vi "String_to_Pathname.vi"(1 "Input String":string) -> (0 "path":path)   [LabVIEW 2014]
uses:
  Globals/Preference_global.vi
  Globals/Constants_global.vi
panel:
  out "size(s)":i32
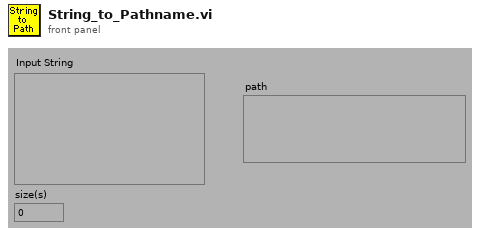
[diagram p1: front panel]
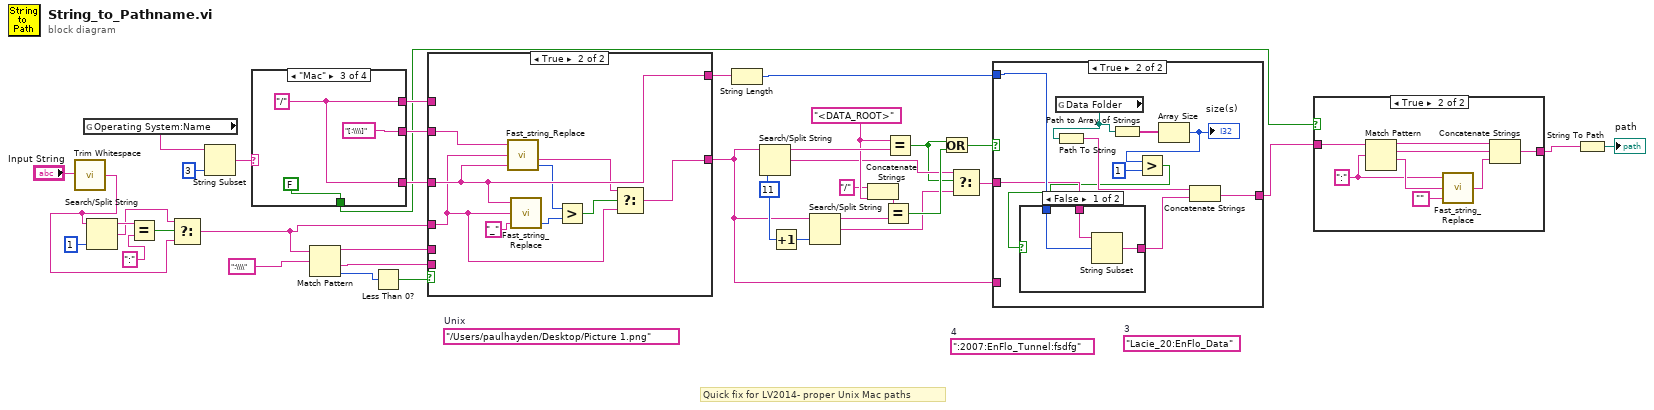
[diagram p0: block diagram]
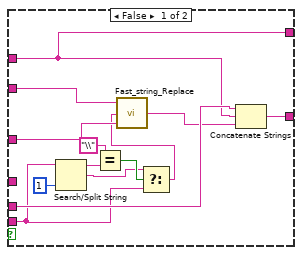
[diagram p5: hidden frame]
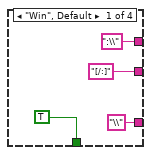
[diagram p6: hidden frame]
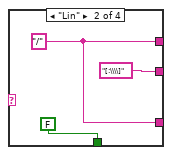
[diagram p7: hidden frame]
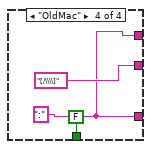
[diagram p8: hidden frame]
diagram:
  (unwired) "Lacie_20:EnFlo_Data"  # 3
  (unwired) ":2007:EnFlo_Tunnel:fsdfg"  # 4
  (unwired) "/Users/paulhayden/Desktop/Picture 1.png"  # Unix
  w13 = 11
  w9 = "<DATA_ROOT>" ("regular expression")
  # "Quick fix for LV2014- proper Unix Mac paths"
  n1 = call <vilib>:"Trim Whitespace.vi"("string"="Input String") -> ("trimmed string"=w17:string)  [unwired: 1 in]
  n2 = global read "Preference_global.vi" "Operating System:Name"() -> (w38:string)
  n3 = Search/Split String(string=w17, offset (0)=1 ("length (rest)")) -> (substring before match=w28:string, match + rest of string=w27:string)  [unwired: 2 out]
  n4 = Equal?(x=w28, y=":") -> (x = y?=w30:bool)
  n5 = Select(t=w27, s=w30, f=w17) -> (s? t:f=w26:string)
  n6 = String Subset(string=w38, length (rest)=3 ("length (rest)")) -> (substring=w39:string)  [unwired: 1 out]
  n7 = case shown="\"Mac\"" w39 {
    tunnel: ["[/:]" "[:\\\\]" "[:\\\\]" "[/\\\\]"] -> w33
    tunnel: ["\\" w45 w48 w51] -> w32
    tunnel: [":\\" w45 w48 w51] -> w21
    tunnel: [TRUE FALSE FALSE FALSE] -> w14
    frame "Win", Default {
    }
    frame "Lin" {
      w45 = "/"
    }
    frame "Mac" {
      w48 = "/"
    }
    frame "OldMac" {
      w51 = ":"
    }
  }
  n8 = Match Pattern(string=w26, regular expression=":\\\\") -> (before substring=w24:string, after substring=w25:string, offset past match=w35:i32)  [unwired: 2 out]
  n9 = Less Than 0?(x=w35) -> (x < 0?=w34:bool)
  n10 = case shown="True" w34 {
    tunnel: w26 -> [_ w67]
    tunnel: w33 -> [w65 w74]
    tunnel: w32 -> [w64 w73]
    tunnel: w25 -> [w54 _]
    tunnel: w24 -> [w63 _]
    tunnel: w21 -> [w60 _]
    tunnel: [w61 w66] -> w5
    tunnel: [w60 w73] -> w19
    frame False {
      n11 = Search/Split String(string=w54, offset (0)=1 ("length (rest)")) -> (substring before match=w58:string, match + rest of string=w55:string)  [unwired: 2 out]
      n12 = Equal?(x="\\", y=w58) -> (x = y?=w56:bool)
      n13 = Select(t=w55, s=w56, f=w54) -> (s? t:f=w53:string)
      n14 = call "Fast_string_Replace.vi"("Replace match with:"=w64, "Input String"=w53, "regular expression"=w65) -> ("Output String"=w62:string)  [unwired: 2 out]
      n15 = Concatenate Strings(w63, w60, w62) -> (w61:string)
    }
    frame True {
      n16 = call "Fast_string_Replace.vi"("Replace match with:"=w73, "Input String"=w67, "regular expression"=w74) -> ("Number Found"=w71:i32, "Output String"=w68:string)  [unwired: 1 out]
      n17 = call "Fast_string_Replace.vi"("Replace match with:"="_", "Input String"=w67, "regular expression"=w73) -> ("Number Found"=w70:i32)  [unwired: 2 out]
      n18 = Greater?(x=w71, y=w70) -> (0:w69:bool)
      n19 = Select(t=w68, s=w69, f=w67) -> (s? t:f=w66:string)
    }
  }
  n20 = String Length(string=w19) -> (length=w20:i32)
  n21 = Search/Split String(string=w5, offset (0)=w13) -> (substring before match=w23:string, match + rest of string=w2:string)  [unwired: 1 in, 1 out]
  n22 = Increment(x=w13) -> (x+1=w12:i32)
  n23 = Search/Split String(string=w5, offset (0)=w12) -> (substring before match=w11:string, match + rest of string=w3:string)  [unwired: 1 in, 1 out]
  n24 = Concatenate Strings("/" ("string"), w9) -> (w10:string)
  n25 = Equal?(x=w10, y=w11) -> (x = y?=w6:bool)
  n26 = Equal?(x=w9, y=w23) -> (x = y?=w1:bool)
  n27 = Or(x=w1, y=w6) -> (x .or. y?=w7:bool)
  n28 = Select(t=w2, s=w1, f=w3) -> (s? t:f=w4:string)
  n29 = case shown="True" w7 {
    tunnel: w5 -> [w75 _]
    tunnel: [w75 w79] -> w16
    tunnel: w4 -> [_ w83]
    tunnel: w20 -> [_ w84]
    frame False {
    }
    frame True {
      n30 = global read "Constants_global.vi" "Data Folder"() -> (w81:path)
      n31 = Path To String(path=w81) -> (string=w85:string)
      n32 = Path to Array of Strings(0:w81) -> (2:w80:string[])  [unwired: 1 out]
      n33 = Array Size(array=w80) -> (size(s)=w78:i32)
      "size(s)" <- w78
      n34 = Greater?(x=w78, y=1) -> (0:w76:bool)
      n35 = case shown="False" w76 {
        tunnel: w84 -> [w88 _]
        tunnel: w83 -> [w87 w89]
        tunnel: [w86 w89] -> w82
        frame False {
          n36 = String Subset(string=w87, offset (0)=w88) -> (substring=w86:string)  [unwired: 1 out]
        }
        frame True {
        }
      }
      n37 = Concatenate Strings(w85, w82) -> (w79:string)
    }
  }
  n38 = case shown="True" w14 {
    tunnel: w16 -> [w90 w98]
    tunnel: [w90 w91] -> w15
    frame False {
    }
    frame True {
      w96 = ":" ("regular expression")
      n39 = Match Pattern(string=w98, regular expression=w96) -> (before substring=w93:string, match substring=w92:string, after substring=w97:string)  [unwired: 2 out]
      n40 = call "Fast_string_Replace.vi"("Replace match with:"="", "Input String"=w97, "regular expression"=w96) -> ("Output String"=w94:string)  [unwired: 2 out]
      n41 = Concatenate Strings(w93, w92, w94) -> (w91:string)
    }
  }
  n42 = String To Path(string=w15) -> (path=→"path":path)
